vi "VI Reference AE.vi"(7 "error in":errorcluster, 9 "Main VI Path":path, 10 "Action":T2=enum."Create") -> (0 "error out":errorcluster, 3 "Master Reference":T1)   [LabVIEW 2024, in "Copia Exacta de Clon.lvlib" / "VI Reference Management.lvlib"]
doc: "A functional global (implemented as an Action Engine) used to store the master VI reference for spawning instances of the cloneable Main VI. \n_____\nBased on DQMH Dev Tools: Project Template 7.1.0.1503."
uses:
  VI Reference Management.lvlib
  Action--enum.ctl
  Main VI Type--strict_vi_ref.ctl
  <vilib>/Delacor/Delacor QMH/Libraries/Cloneable Module Admin_class/Delacor_lib_QMH_Cloneable Module Admin.lvclass
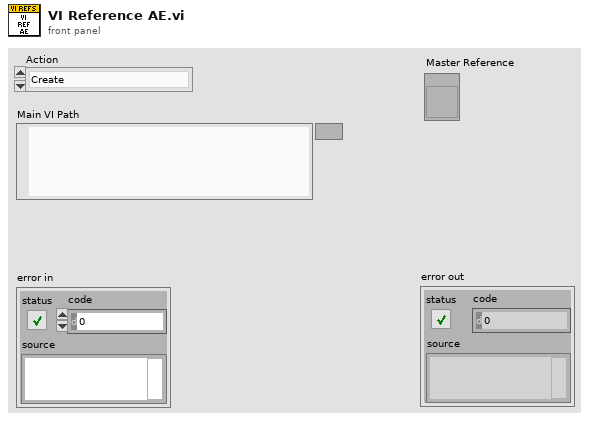
[diagram p1: front panel]
types:
  T1 = typedef "Copia Exacta de Clon.lvlib/VI Reference Management.lvlib/Main VI Type--strict_vi_ref.ctl" = refnum<vi>
  T2 = typedef "Copia Exacta de Clon.lvlib/VI Reference Management.lvlib/Action--enum.ctl" = enum16{"Get", "Create", "Close"}
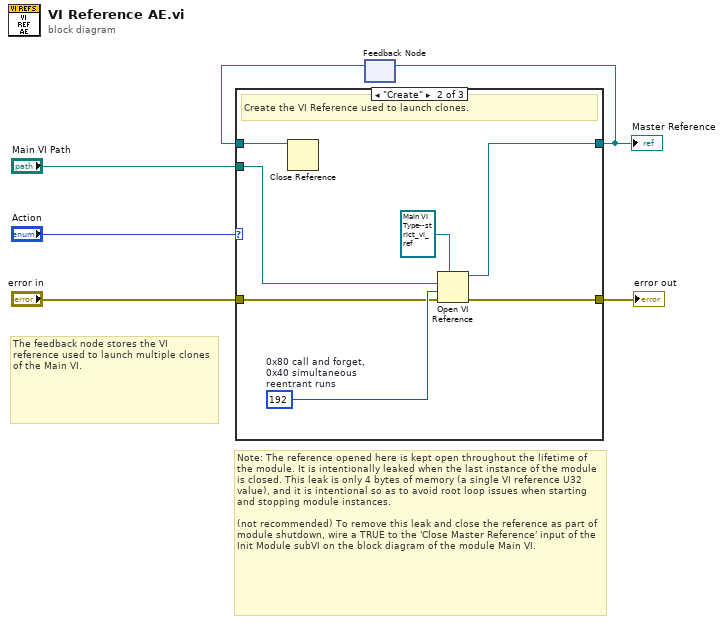
[diagram p0: block diagram]
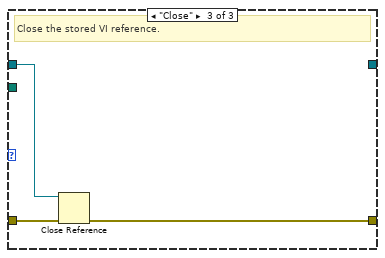
[diagram p3: hidden frame]
diagram:
  # "Note: The reference opened here is kept open throughout the lifetime of the module. It is intentionally leaked when the last instance of the module is closed. This leak is only 4 bytes of memory (a single VI reference U32 value), and it is intentional so as to avoid root loop issues when starting and stopping module instances.\n\n(not recommended) To remove this leak and close the reference as part of module shutdown, wire a TRUE to the 'Close Master Reference' input of the Init Module subVI on the block diagram of the module Main VI."
  # "The feedback node stores the VI reference used to launch multiple clones of the Main VI."
  n1 = feedback #1() -> (w5:T1)  [unwired: 1 in]
  n2 = case shown="\"Create\"" "Action" {
    tunnel: w5 -> [w7 w9 w16]
    tunnel: [w7 w10 _] -> w1
    tunnel: "error in" -> [w8 w13 w18]
    tunnel: [w8 w11 w17] -> w3
    tunnel: "Main VI Path" -> [_ w12 _]
    frame "Get" {
      # "Get the current VI reference"
    }
    frame "Create" {
      w15 = 192  # 0x80 call and forget, 0x40 simultaneous reentrant runs
      # "Create the VI Reference used to launch clones."
      n3 = Close Reference(reference=w9) -> ()  [unwired: 1 in, 1 out]
      n4 = Open VI Reference(type specifier VI Refnum (for type only)=T1 refnum ("Main VI Type"), vi path=w12, options=w15, error in (no error)=w13) -> (vi reference=w10:T1, error out=w11:errorcluster)  [unwired: 2 in]
    }
    frame "Close" {
      # "Close the stored VI reference."
      n5 = Close Reference(reference=w16, error in (no error)=w18) -> (error out=w17:errorcluster)
    }
  }
  "error out" <- w3
  "Master Reference" <- w1
  n6 = feedback-in #1(w1) -> ()
